vi "Dashboard Main.vi"() -> ()   [LabVIEW 2012]
uses:
  <vilib>/event_ctls.llb/eventvkey.ctl
  <vilib>/Utility/config.llb/Read Key (String).vi
  <vilib>/Utility/config.llb/Read Key (I32).vi
  <vilib>/Utility/config.llb/Write Key (String).vi
  <vilib>/Utility/config.llb/Write Key (I32).vi
  <vilib>/Utility/config.llb/NI_LVConfig.lvlib
panel:
  out "Decal 25":bool
  out "Decal 24":bool
  out "Decal 23":bool
  out "Decal 22":bool
  out "Decal 21":bool
  out "Decal 20":bool
  out "Decal 19":bool
  out "Decal 18":bool
  out "Decal 17":bool
  out "Decal 16":bool
  out "Decal 15":bool
  out "Decal 14":bool
  out "Decal 13":bool
  out "Decal 12":bool
  out "Decal 11":bool
  out "Decal 10":bool
  out "Decal 9":bool
  out "Decal 8":bool
  out "Decal 7":bool
  out "Decal 6":bool
  out "Decal 5":bool
  out "Decal 4":bool
  out "Decal 3":bool
  out "Decal 2":bool
  out "Decal 1":bool
  in  "Camera Settings":T1={"Frate Rate"=30, "Compression"=30, "Size"=1} {"Frate Rate" scale=1.0..30.0; "Size" items=["640x480", "320x240", "160x120"]}
  out "Mode":T2(ring)=enum."Auto Disabled"
  out "Camera IP":string
  in  "Dashboard Tab":enum32{"Operation", "Test", "Checklist"}(tab)
  out "Height":dbl format="%#_4g"
  out "Move Y":dbl format="%#_4g"
  out "Move X":dbl format="%#_4g"
  out "Rotation":dbl format="%#_4g"
  out "Min Height":bool
  out "Max Height":bool
  out "Feed Disc":bool
  in  "Set Launcher":dbl(slide) scale=0.0..100.0
  in  "Invert Motors":bool
  out "Rotation Output":dbl(knob) scale=0.0..100.0
  out "Linear Output":dbl(knob) scale=0.0..100.0
  out "Launcher Power":dbl(knob) scale=0.0..100.0
  out "Low Battery":bool
  out "FMS":bool
  out "Test":bool
  out "Teleop":bool
  out "Auto":bool
  out "Disabled":bool
  out "Program:":string caption="Program"
  out "Robot IP:":string caption="Robot IP"
  in  "Slider":dbl(slide) scale=0.0..100.0 scale format="%#_3g"
  in  "On/Off":bool caption="Solenoid"
  in  "Test Name":u16(ring) items=["Select the test to run...", "Example Test", "-------------------------------", "List of tests is built in robot code.", "Replace with your own automated tests."]
  in  "Test Tree":string(tree)
  in  "Motor":cluster{"Value":dbl, "Enable":bool} {"Value" scale=-1.0..1.0 scale format="%#_3g"}
  out "Progress":T3 {"Test Progress" scale=0.0..100.0}
  in  "Rev/Fwd":cluster{"Forward":bool, "Reverse":bool}
  in  "Ring":u16(ring) items=["Auto", "Fixed indoor", "Fixed outdoor 1", "Fixed outdoor 2", "Fixed fluorescent 1", "Fixed fluorescent 2", "Hold current"]
  in  "Listbox":i32(listbox)
  in  "Viewer":enum32{"Camera Image", "Variables"}(tab)
  in  "DB Camera Config":bool
  out "Mbps":dbl format="%#.1g"
  out "Mbps":bool
  in  "Enable":bool
  out "Image Error Message":string="Timeout in Camera Communications"
  out "Camera Image":T4(plugin-control)
  out "Tree":string(tree)
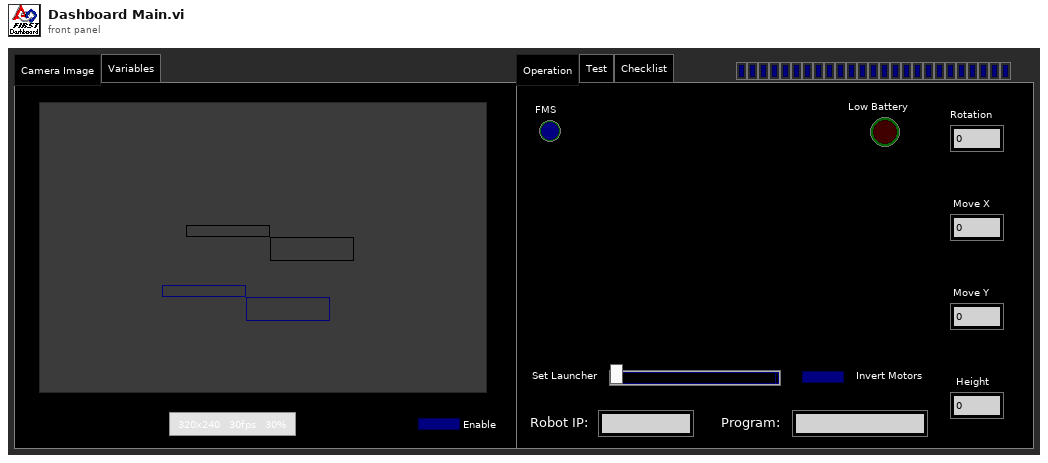
[diagram p1: front panel]
types:
  T1 = cluster{"Frate Rate":i32, "Compression":i32, "Size":u16}
  T2 = enum8{"Tele-Op Disabled", "Tele-Op Enabled", "Auto Disabled", "Auto Enabled", "Test Disabled", "Test Enabled", ""}
  T3 = cluster{"Test Progress":u8, "Test Progress Text":string}
  T4 = typedef "IMAQ Image.ctl" = refnum<image>
  T5 = typedef "Image Type" = u32
  T6 = typedef "SkeletonTrackState.ctl" = enum32{"NotTracked", "PositionOnly", "Tracked"}
  T7 = cluster{"TrackingState":u8[], "Position":cluster{"x":sgl, "y":sgl, "z":sgl}, cluster{"x":sgl, "y":sgl, "z":sgl, sgl}[], "TrackState":T6}
  T8 = cluster{cluster{"ScaledToPercentRange":dbl, "ScaledToPercentRange":dbl, "ScaledToPercentRange":dbl}, cluster{bool, bool, bool}}[]
  T9 = cluster{cluster{"ScaledToPercentRange":dbl, "ScaledToPercentRange":dbl, "ScaledToPercentRange":dbl}, cluster{bool, bool, bool}}
  T10 = typedef "LVRectTypeDef.ctl" = cluster{"Left":i16, "Top":i16, "Right":i16, "Bottom":i16}
  T11 = cluster{"Competition mode":bool, "Robot Link":bool, "Autonomous":bool, "Enabled":bool, "E-Stop":bool, "Simulated":bool, "TestMode":bool, "Docked Window":bool}
  T12 = typedef "NI_LVConfig.lvlib/Config Data RefNum.ctl" = refnum<k1>
  T13 = typedef "eventvkey.ctl" = enum16{"ASCII", "Enter", "Return", "Shift", "Ctrl", "Alt", "Cmd", "Opt", "Caps", "NumLock", "Clear", "Break", "Up", "Down", "Left", "Right", "Insert", "Delete", "Home", "End", "PageUp", "PageDown", "Escape", "Help", "Pause", "ScrollLock", "F1", "F2", "F3", "F4", "F5", "F6", "F7", "F8", "F9", "F10", "F11", "F12", "F13", "F14", "F15", "F16", "F17", "F18", "F19", "F20", "F21", "F22", "F23", "F24", "Play", "VolumeUp", "VolumeDown", "Mute", "Two Byte Char"}
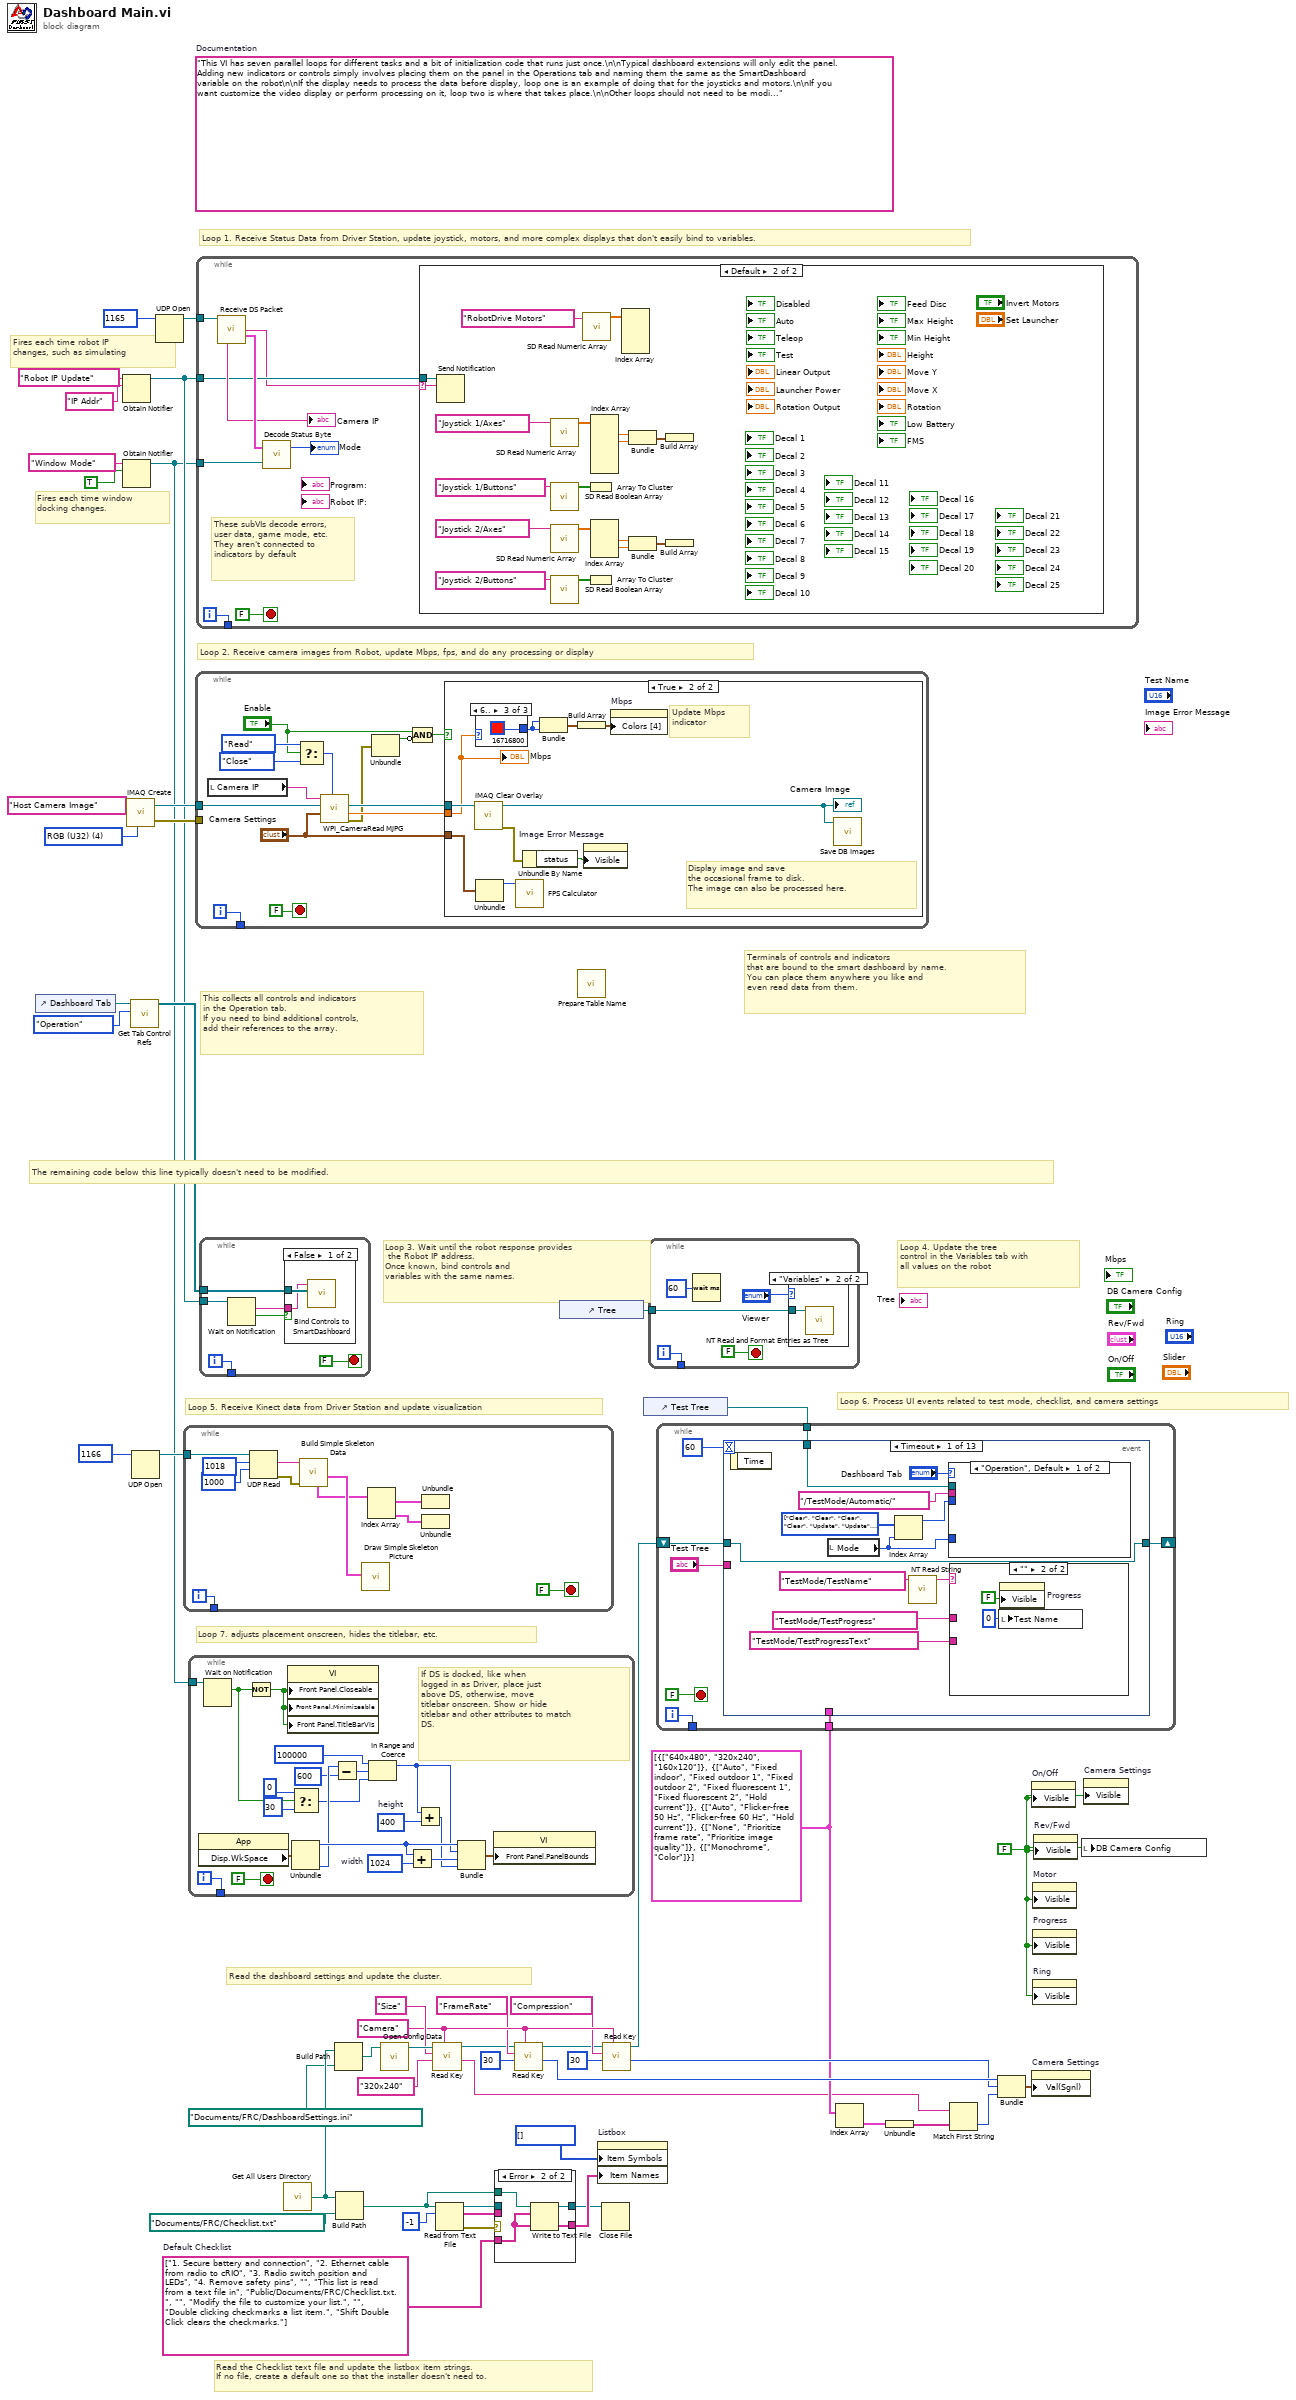
[diagram p0: block diagram]
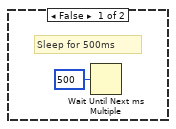
[diagram p3: hidden frame]
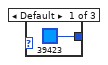
[diagram p4: hidden frame]
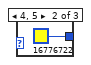
[diagram p5: hidden frame]
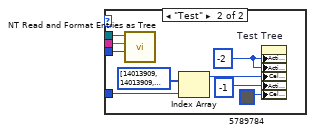
[diagram p7: hidden frame]
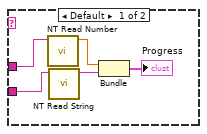
[diagram p8: hidden frame]
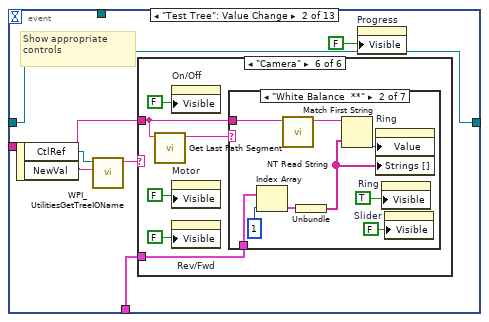
[diagram p9: hidden frame]
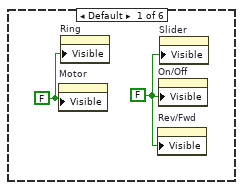
[diagram p10: hidden frame]
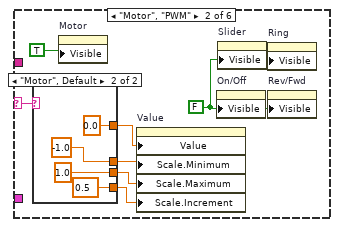
[diagram p11: hidden frame]
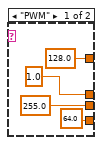
[diagram p12: hidden frame]
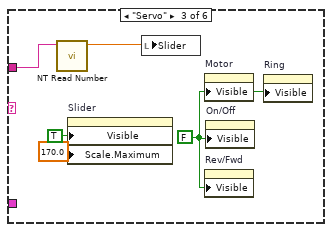
[diagram p13: hidden frame]
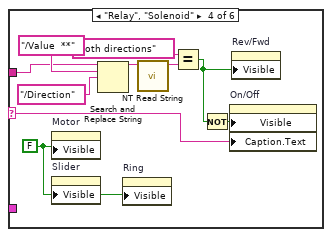
[diagram p14: hidden frame]
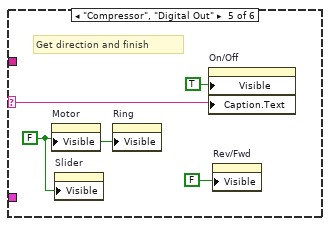
[diagram p15: hidden frame]
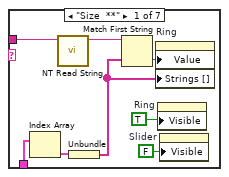
[diagram p16: hidden frame]
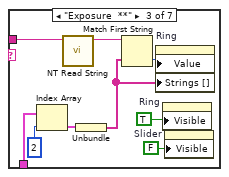
[diagram p17: hidden frame]
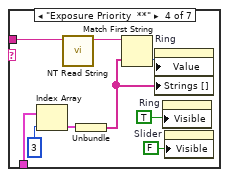
[diagram p18: hidden frame]
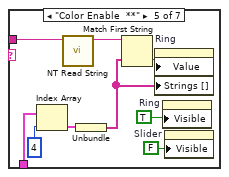
[diagram p19: hidden frame]
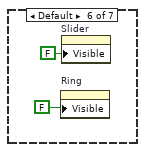
[diagram p20: hidden frame]
diagram:
  w21 = "Camera"
  w13 = cluster{string[]}[] [{["640x480", "320x240", "160x120"]}, {["Auto", "Fixed indoor", "Fixed outdoor 1", "Fixed outdoor 2", "Fixed fluorescent 1", "Fixed fluorescent 2", "Hold current"]}, {["Auto", "Flicker-free 50 Hz", "Flicker-free 60 Hz", "Hold current"]}, {["None", "Prioritize frame rate", "Prioritize image quality"]}, {["Monochrome", "Color"]}]
  w29 = string[] ["1. Secure battery and connection", "2. Ethernet cable from radio to cRIO", "3. Radio switch position and LEDs", "4. Remove safety pins", "", "This list is read from a text file in", "Public/Documents/FRC/Checklist.txt.", "", "Modify the file to customize your list.", "", "Double clicking checkmarks a list item.", "Shift Double Click clears the checkmarks."]  # Default Checklist
  w27 = FALSE ("Visible")
  (unwired) "This VI has seven parallel loops for different tasks and a bit of initialization code that runs just once.\n\nTypical dashboard extensions will only edit the panel. Adding new indicators or controls simply involves placing them on the panel in the Operations tab and naming them the same as the SmartDashboard variable on the robot\n\nIf the display needs to process the data before display, loop one is an example of doing that for the joysticks and motors.\n\nIf you want customize the video display or perform processing on it, loop two is where that takes place.\n\nOther loops should not need to be modified. They are pretty standard, and document the task they perform."  # Documentation
  w50 = T5 4 items=["Grayscale (U8)", "Grayscale (I16)", "Grayscale (SGL)", "Complex (CSG)", "RGB (U32)", "HSL (U32)", "RGB (U64)"] ("Image Type")
  # "Fires each time robot IP\nchanges, such as simulating"
  # "Fires each time window\ndocking changes."
  # "Read the Checklist text file and update the listbox item strings.\nIf no file, create a default one so that the installer doesn't need to."
  # "This collects all controls and indicators\nin the Operation tab.\nIf you need to bind additional controls,\nadd their references to the array."
  # "The remaining code below this line typically doesn't need to be modified."
  # "Loop 6. Process UI events related to test mode, checklist, and camera settings"
  # "Read the dashboard settings and update the cluster."
  # "Terminals of controls and indicators\nthat are bound to the smart dashboard by name.\nYou can place them anywhere you like and\neven read data from them."
  # "Loop 4. Update the tree\ncontrol in the Variables tab with\nall values on the robot"
  # "Loop 3. Wait until the robot response provides\n the Robot IP address.\nOnce known, bind controls and\nvariables with the same names."
  # "Loop 5. Receive Kinect data from Driver Station and update visualization"
  # "Loop 7. adjusts placement onscreen, hides the titlebar, etc."
  # "Loop 1. Receive Status Data from Driver Station, update joystick, motors, and more complex displays that don't easily bind to variables."
  # "Loop 2. Receive camera images from Robot, update Mbps, fps, and do any processing or display"
  n1 = control-ref of="Dashboard Tab"() -> (w43:refnum<vi>)
  n2 = Obtain Notifier(name (unnamed)="Robot IP Update", notification data type="IP Addr" ("name (unnamed)")) -> (notifier out=w40:refnum<notifier>)  [unwired: 2 in, 2 out]
  n3 = Obtain Notifier(name (unnamed)="Window Mode", notification data type=TRUE) -> (notifier out=w33:refnum<notifier>)  [unwired: 2 in, 2 out]
  n4 = call "IMAQ Create"("Image Name"="Host Camera Image", "Image Type"=w50) -> ("New Image"=w48:T4, "error out"=w47:errorcluster)  [unwired: 2 in, 1 out]
  n5 = call <vilib>:"Get Tab Control Refs.vi"("Page Index"=enum32{"Operation", "Test"}."Operation" ("Dashboard Tab"), "TabControl in"=w43) -> ("ControlsOnPage"=w44:refnum<vi>[])  [unwired: 9 in]
  n6 = UDP Open(11:u16 1166 ("port")) -> (port=w45:refnum<k16>)  [unwired: 2 in, 4 out]
  n7 = UDP Open(11:u16 1165 ("port")) -> (port=w51:refnum<k16>)  [unwired: 2 in, 4 out]
  n8 = while {
    tunnel: w45 -> [w61]
    tunnel: [w54] -> _
    i -> [w54]
    stop <- FALSE stop-if-true
    n9 = UDP Read(connection ID=w61, max size (548)=1018 ("bytes to read"), timeout ms (25000)=1000) -> (data out=w59:string, error out=w53:errorcluster)  [unwired: 1 in, 3 out]
    n10 = call "Build Simple Skeleton Data.vi"("error in (no error)"=w53, "data in"=w59) -> ("Skeleton Data"=w60:T7, "Simple Joystick Info"=w57:T8)  [unwired: 5 in, 3 out]
    n11 = call "Draw Simple Skeleton Picture.vi"("Simple Skeleton"=w60) -> ()  [unwired: 10 in, 1 out]
    n12 = Index Array(array=w57) -> (element #1=w56:T9, element #2=w55:T9)  [unwired: 2 in]
    n13 = Unbundle(w56) -> ()  [unwired: 2 out]
    n14 = Unbundle(w55) -> ()  [unwired: 2 out]
  }
  n15 = while {
    tunnel: w33 -> [w82]
    tunnel: [w80] -> _
    i -> [w80]
    stop <- FALSE stop-if-true
    w72 = 1024  # width
    w75 = 400  # height
    # "If DS is docked, like when\nlogged in as Driver, place just\nabove DS, otherwise, move\ntitlebar onscreen. Show or hide\ntitlebar and other attributes to match\nDS."
    n16 = property class="App"() -> ("Disp.WkSpace"=w78:T10)  [unwired: 2 in, 2 out]
    n17 = Wait on Notification(notifier=w82) -> (notification=w67:bool)  [unwired: 3 in, 3 out]
    n18 = Not(x=w67) -> (.not. x?=w81:bool)
    n19 = property class="VI"("Front Panel.Closeable"=w81, "Front Panel.Minimizeable"=w81, "Front Panel.TitleBarVis"=w81) -> ()  [unwired: 2 in, 2 out]
    n20 = Unbundle(w78) -> ("Left"=w76:i16, "Bottom"=w73:i16)  [unwired: 2 out]
    n21 = Select(t=0, s=w67, f=30) -> (s? t:f=w66:i32)
    n22 = Subtract(x=w73, y=600) -> (x-y=w70:i32)
    n23 = In Range and Coerce(upper limit=100000, x=w70, lower limit=w66) -> (coerced(x)=w64:i32)  [unwired: 1 out]
    n24 = Add(x=w76, y=w72) -> (x+y=w77:i32)
    n25 = Add(x=w64, y=w75) -> (x+y=w74:i32)
    n26 = Bundle("Left"=w76, w64, w77, w74) -> (w79:cluster{"Left":i16, i32, i32, i32})  [unwired: 1 out]
    n27 = property class="VI"("Front Panel.PanelBounds"=w79) -> ()  [unwired: 2 in, 2 out]
  }
  n28 = while {
    tunnel: w48 -> [w93]
    tunnel: w47 -> [_]
    tunnel: [w96] -> _
    i -> [w96]
    stop <- FALSE stop-if-true
    n29 = local read "Camera IP"() -> (w95:string)
    n30 = Select(t=enum16{"Read", "Reopen", "Close"}."Read" ("Operation"), s="Enable", f=enum16{"Read", "Reopen", "Close"}."Close" ("Operation")) -> (s? t:f=w88:enum16{"Read", "Reopen", "Close"})
    n31 = call <vilib>:"WPI_CameraRead MJPG.vi"("Operation"=w88, "Camera Settings"="Camera Settings", "Image"=w93, "address"=w95) -> ("error out"=w87:errorcluster, "Bandwidth (kbps)"=w91:dbl, "Image Out"=w92:T4)  [unwired: 5 in]
    n32 = Unbundle(w87) -> ("status"=w85:bool)  [unwired: 2 out]
    n33 = Compound Arithmetic op=AND("Enable", invert w85) -> (w84:bool)
    n34 = case shown="True" w84 {
      tunnel: "Camera Settings" -> [_ w100]
      tunnel: w92 -> [_ w102]
      tunnel: w91 -> [_ w101]
      frame False {
        # "Sleep for 500ms"
        n35 = Wait Until Next ms Multiple(millisecond multiple=u32 500) -> ()  [unwired: 1 out]
      }
      frame True {
        # "Display image and save\nthe occasional frame to disk.\nThe image can also be processed here."
        # "Update Mbps\nindicator"
        n36 = call "IMAQ Clear Overlay"("Image"=w102) -> ("error out"=w107:errorcluster, "Image Out"=w106:T4)  [unwired: 2 in, 7 out]
        "Camera Image" <- w106
        n37 = case shown="6.." w101 {
          tunnel: [u32 39423 ("Color Box") u32 16776722 ("Color Box") u32 16716800 ("Color Box")] -> w103
          frame Default {
          }
          frame 4, 5 {
          }
          frame 6.. {
          }
        }
        n38 = Unbundle(w100) -> ("Frate Rate"=w99:i32)  [unwired: 2 out]
        n39 = call "FPS Calculator.vi"("Average Count"=w99) -> ()  [unwired: 10 in, 1 out]
        n40 = Unbundle By Name(w107) -> ("status"=w108:bool)
        n41 = Bundle("Color Box"=w103, "Color Box"=w103) -> (w105:cluster{"Color Box":u32, "Color Box":u32})  [unwired: 1 out]
        n42 = Build Array(w105) -> (w104:cluster{"Color Box":u32, "Color Box":u32}[])
        n43 = property on="Image Error Message" class="Str"("Visible"=w108) -> ()  [unwired: 2 in, 2 out]
        n44 = property on="Mbps" class="Bool (strict)"("Colors [4]"=w104) -> ()  [unwired: 2 in, 2 out]
        n45 = call "Save DB Images.vi"("Image"=w106) -> ()  [unwired: 2 in, 1 out]
        "Mbps" <- w101
      }
    }
  }
  n46 = while {
    tunnel: w51 -> [w118]
    tunnel: w40 -> [w113]
    tunnel: w33 -> [w117]
    tunnel: [w114] -> _
    i -> [w114]
    stop <- FALSE stop-if-true
    # "These subVIs decode errors, user data, game mode, etc.\nThey aren't connected to indicators by default"
    n47 = call "Receive DS Packet.vi"("Recv Socket"=w118) -> ("Robot IP Address"=w112:string, "Status"=w119:T11, "Camera IP Address"=→"Camera IP":string)  [unwired: 1 in, 11 out]
    n48 = call "Decode Status Byte.vi"("Window Mode Notifier"=w117, "Status"=w119) -> ("Mode"=→"Mode":T2)  [unwired: 1 out]
    n49 = case shown="Default" w112 {
      selector: w112 -> [_ w121]
      tunnel: w113 -> [_ w122]
      frame "0.0.0.0" {
        # "Robot not responding, don't poll the variables"
      }
      frame Default {
        n50 = Send Notification(notification=w121, notifier=w122) -> ()  [unwired: 1 in, 2 out]
        n51 = call <vilib>:"SD Read Numeric Array.vi"("Name"="Joystick 1/Axes") -> ("Numeric Array"=w133:dbl[])  [unwired: 8 in, 2 out]
        n52 = call <vilib>:"SD Read Boolean Array.vi"("Name"="Joystick 1/Buttons") -> ("Boolean Array"=w134:bool[])  [unwired: 8 in, 2 out]
        n53 = call <vilib>:"SD Read Numeric Array.vi"("Name"="Joystick 2/Axes") -> ("Numeric Array"=w129:dbl[])  [unwired: 8 in, 2 out]
        n54 = call <vilib>:"SD Read Boolean Array.vi"("Name"="Joystick 2/Buttons") -> ("Boolean Array"=w128:bool[])  [unwired: 8 in, 2 out]
        n55 = call <vilib>:"SD Read Numeric Array.vi"("Name"="RobotDrive Motors") -> ("Numeric Array"=w135:dbl[])  [unwired: 8 in, 2 out]
        n56 = Array To Cluster(array=w134) -> ()  [unwired: 1 out]
        n57 = Array To Cluster(array=w128) -> ()  [unwired: 1 out]
        n58 = Index Array(array=w133) -> (element #1=w131:dbl, element #2=w132:dbl)  [unwired: 6 in, 4 out]
        n59 = Index Array(array=w129) -> (element #1=w124:dbl, element #2=w123:dbl)  [unwired: 3 in, 1 out]
        n60 = Index Array(array=w135) -> ()  [unwired: 4 in, 4 out]
        n61 = Bundle("Numeric"=w131, "Numeric"=w132) -> (w130:cluster{"Numeric":dbl, "Numeric":dbl})  [unwired: 1 in]
        n62 = Bundle("Numeric"=w124, "Numeric"=w123) -> (w125:cluster{"Numeric":dbl, "Numeric":dbl})  [unwired: 1 in]
        n63 = Build Array(w130) -> ()  [unwired: 1 out]
        n64 = Build Array(w125) -> ()  [unwired: 1 out]
      }
    }
  }
  n65 = while {
    tunnel: w44 -> [w144]
    tunnel: w40 -> [w141]
    tunnel: [w139] -> _
    i -> [w139]
    stop <- FALSE stop-if-true
    n66 = Wait on Notification(notifier=w141) -> (notification=w140:string, timed out?=w142:bool)  [unwired: 3 in, 2 out]
    n67 = case shown="False" w142 {
      tunnel: w144 -> [w146 _]
      tunnel: w140 -> [w145 _]
      frame False {
        n68 = call <vilib>:"Bind Controls to SmartDashboard.vi"("Bound Control Refs"=w146, "Server IP Address"=w145) -> ()  [unwired: 10 in]
      }
      frame True {
      }
    }
  }
  n69 = call "Get All Users Directory.vi"() -> ("All User Path"=w26:path)
  n70 = Build Path(base path=w26, name or relative path=path "Documents/FRC/DashboardSettings.ini") -> (appended path=w25:path)
  n71 = Build Path(base path=w26, name or relative path=path "Documents/FRC/Checklist.txt") -> (appended path=w30:path)
  n72 = call <vilib>:"Open Config Data.vi"("configuration file path"=w25) -> ("refnum"=w24:T12)  [unwired: 8 in, 2 out]
  n73 = call-poly <vilib>:"Read Key.vi"("section"=w21, "default value"="320x240", "key"="Size", "refnum"=w24) -> ("value"=w11:string, "refnum out"=w6:T12)  [unwired: 2 in, 4 out]
  n74 = Read from Text File(file (use dialog)=w30, count=-1 ("timeout ms (25000)")) -> (refnum out=w8:refnum<file>, text=w31:string[], error out=w32:errorcluster)  [unwired: 2 in, 1 out]
  n75 = case shown="Error" w32 {
    tunnel: w31 -> [w148 _]
    tunnel: [w148 w150] -> w28
    tunnel: w29 -> [_ w150]
    tunnel: w30 -> [_ w151]
    tunnel: [w147 w149] -> w7
    tunnel: w8 -> [w147 _]
    frame No Error {
    }
    frame Error {
      n76 = Write to Text File(file (use dialog)=w151, text=w150) -> (refnum out=w149:refnum<file>)  [unwired: 2 in, 2 out]
    }
  }
  n77 = call-poly <vilib>:"Read Key.vi"("section"=w21, "default value"=30, "key"="FrameRate", "refnum"=w6) -> ("value"=w16:i32, "refnum out"=w5:T12)  [unwired: 1 in, 5 out]
  n78 = control-ref of="Tree"() -> (w2:refnum<vi>)
  n79 = call <vilib>:"Prepare Table Name.vi"() -> ()  [unwired: 11 in, 1 out]
  n80 = property on="Listbox" class="LstBox (strict)"("Item Symbols"=i32[] [], "Item Names"=w28) -> ()  [unwired: 2 in, 2 out]
  n81 = Close File(refnum=w7) -> ()  [unwired: 1 in, 2 out]
  n82 = call-poly <vilib>:"Read Key.vi"("section"=w21, "default value"=30, "key"="Compression", "refnum"=w5) -> ("value"=w15:i32, "refnum out"=w3:T12)  [unwired: 1 in, 5 out]
  n83 = control-ref of="Test Tree"() -> (w1:refnum<vi>)
  n84 = while {
    tunnel: [w153] -> _
    tunnel: w2 -> [w152]
    i -> [w153]
    stop <- FALSE stop-if-true
    n85 = Wait (ms)(milliseconds to wait=u32 60) -> ()  [unwired: 1 out]
    n86 = case shown="\"Variables\"" "Viewer" {
      tunnel: w152 -> [_ w157]
      frame Default {
      }
      frame "Variables" {
        n87 = call <vilib>:"NT Read and Format Entries as Tree.vi"("Tree Refnum"=w157) -> ()  [unwired: 9 in, 2 out]
      }
    }
  }
  n88 = while {
    tunnel: w13 -> [w162]
    shift-right: [w161] -> _
    shift-left: w3 -> [w160]
    tunnel: [w159] -> _
    tunnel: w1 -> [w158]
    i -> [w159]
    stop <- FALSE stop-if-true
    n89 = event shown="[0] Timeout" {
      selector: _ -> [_ _ _ _ _ _ _ _ _ _ _ _ _]
      dyn-events: _ -> [_ _ _ _ _ _ _ _ _ _ _ _ _]
      timeout: u32 60 ("milliseconds to wait") -> [_ _ _ _ _ _ _ _ _ _ _ _ _]
      tunnel: w158 -> [w172 _ _ _ _ _ _ _ _ _ _ _ _]
      tunnel: "Test Tree" -> [_ _ _ _ _ _ _ _ w366 w374 w376 w380 w388]
      tunnel: w162 -> [_ w194 _ _ _ _ w330 w360 _ _ _ _ _]
      tunnel: [w166 w193 _ w296 w304 w316 w329 w353 w365 w372 w375 w379 w387] -> w161
      tunnel: w160 -> [w166 w193 _ w296 w304 w316 w328 w353 w365 w372 w375 w379 w387]
      event Timeout {
        w171 = enum16{"Update", "Clear"}[] [enum."Clear", enum."Clear", enum."Clear", enum."Clear", enum."Update", enum."Update", enum."Clear"] items=["Update", "Clear"]
        n90 = event-data() -> ()  [unwired: 1 in, 1 out]
        n91 = local read "Mode"() -> (w169:T2)
        n92 = Index Array(array=w171, index=w169) -> (element=w170:enum16{"Update", "Clear"})
        n93 = call <vilib>:"NT Read String.vi"("Name"="TestMode/TestName") -> ("String"=w175:string)  [unwired: 9 in, 1 out]
        n94 = case shown="\"Operation\", Default" "Dashboard Tab" {
          tunnel: w172 -> [_ w185]
          tunnel: "/TestMode/Automatic/" ("Name Pattern") -> [_ w184]
          tunnel: w170 -> [_ w183]
          tunnel: w169 -> [_ w181]
          frame "Operation", Default {
          }
          frame "Test" {
            w180 = -2 ("Active Item:Row Number")
            n95 = call <vilib>:"NT Read and Format Entries as Tree.vi"("Operation"=w183, "Name Pattern"=w184, "Tree Refnum"=w185) -> ()  [unwired: 7 in, 2 out]
            n96 = Index Array(array=u32[] [14013909, 14013909, 14013909, 14013909, 14013909, 16777215, 14013909], index=w181) -> (element=w179:u32)
            n97 = property on="Test Tree" class="Tree (strict)"("Active Item Row Number"=w180, "ActiveColNum"=w180, "CellBG"=w179, "Active Item Row Number"=-1 ("Active Item:Row Number"), "CellBG"=u32 5789784 ("Color Box")) -> ()  [unwired: 2 in, 2 out]
          }
        }
        n98 = case shown="\"\"" w175 {
          tunnel: "TestMode/TestProgress" ("Name") -> [w187 _]
          tunnel: "TestMode/TestProgressText" ("Name") -> [w186 _]
          frame Default {
            n99 = call <vilib>:"NT Read Number.vi"("Name"=w187) -> ("Numeric"=w188:dbl)  [unwired: 9 in, 1 out]
            n100 = call <vilib>:"NT Read String.vi"("Name"=w186) -> ("String"=w189:string)  [unwired: 9 in, 1 out]
            n101 = Bundle("Numeric"=w188, "String"=w189) -> (→"Progress":cluster{"Numeric":dbl, "String":string})  [unwired: 1 in]
          }
          frame "" {
            n102 = local write "Test Name"(u16 0) -> ()
            n103 = property on="Progress" class="Clust (strict)"("Visible"=FALSE) -> ()  [unwired: 2 in, 2 out]
          }
        }
      }
      event "Test Tree": Value Change {
        # "Show appropriate\ncontrols"
        n104 = event-data() -> ("CtlRef"=w197:refnum<vi>, "NewVal"=w195:string)  [unwired: 1 in]
        n105 = call <vilib>:"WPI_UtilitiesGetTreeIOName.vi"("NewVal"=w195, "TreeControl in"=w197) -> ("I/O Name"=w198:string)  [unwired: 9 in]
        n106 = case shown="\"Camera\"" w198 {
          selector: w198 -> [_ w205 _ w223 w232 _]
          tunnel: w195 -> [_ _ w220 w222 _ w239]
          tunnel: w194 -> [_ _ _ _ _ w238]
          frame Default {
            w200 = FALSE ("Visible")
            w199 = FALSE ("Visible")
            n107 = property on="Motor" class="Clust (strict)"("Visible"=w199) -> ()  [unwired: 2 in, 2 out]
            n108 = property on="Ring" class="Ring (strict)"("Visible"=w199) -> ()  [unwired: 2 in, 2 out]
            n109 = property on="Rev/Fwd" class="Clust (strict)"("Visible"=w200) -> ()  [unwired: 2 in, 2 out]
            n110 = property on="On/Off" class="Bool (strict)"("Visible"=w200) -> ()  [unwired: 2 in, 2 out]
            n111 = property on="Slider" class="Slide (strict)"("Visible"=w200) -> ()  [unwired: 2 in, 2 out]
          }
          frame "Motor", "PWM" {
            w206 = FALSE ("Visible")
            n112 = case shown="\"Motor\", Default" w205 {
              tunnel: [1.0 ("Value") -1.0 ("Value")] -> w204
              tunnel: [255.0 ("Value") 1.0 ("Value")] -> w203
              tunnel: [128.0 ("Value") 0.0 ("Value")] -> w202
              tunnel: [64.0 ("Value") 0.5 ("Value")] -> w201
              frame "PWM" {
              }
              frame "Motor", Default {
              }
            }
            n113 = property on="Motor" class="Clust (strict)"("Visible"=TRUE) -> ()  [unwired: 2 in, 2 out]
            n114 = property on="Value" class="Slide (strict)"("Value"=w202, "Scale.Minimum"=w204, "Scale.Maximum"=w203, "Scale.Increment"=w201) -> ()  [unwired: 2 in, 2 out]
            n115 = property on="On/Off" class="Bool (strict)"("Visible"=w206) -> ()  [unwired: 2 in, 2 out]
            n116 = property on="Slider" class="Slide (strict)"("Visible"=w206) -> ()  [unwired: 2 in, 2 out]
            n117 = property on="Ring" class="Ring (strict)"("Visible"=w206) -> ()  [unwired: 2 in, 2 out]
            n118 = property on="Rev/Fwd" class="Clust (strict)"("Visible"=w206) -> ()  [unwired: 2 in, 2 out]
          }
          frame "Servo" {
            w218 = FALSE ("Visible")
            n119 = call <vilib>:"NT Read Number.vi"("Name"=w220) -> ("Numeric"=w219:dbl)  [unwired: 9 in, 1 out]
            n120 = property on="Slider" class="Slide (strict)"("Visible"=TRUE, "Scale.Maximum"=170.0 ("Scale.Range:Maximum")) -> ()  [unwired: 2 in, 2 out]
            n121 = local write "Slider"(w219) -> ()
            n122 = property on="Motor" class="Clust (strict)"("Visible"=w218) -> ()  [unwired: 2 in, 2 out]
            n123 = property on="Rev/Fwd" class="Clust (strict)"("Visible"=w218) -> ()  [unwired: 2 in, 2 out]
            n124 = property on="On/Off" class="Bool (strict)"("Visible"=w218) -> ()  [unwired: 2 in, 2 out]
            n125 = property on="Ring" class="Ring (strict)"("Visible"=w218) -> ()  [unwired: 2 in, 2 out]
          }
          frame "Relay", "Solenoid" {
            w221 = FALSE ("Visible")
            n126 = property on="Motor" class="Clust (strict)"("Visible"=w221) -> ()  [unwired: 2 in, 2 out]
            n127 = property on="Slider" class="Slide (strict)"("Visible"=w221) -> ()  [unwired: 2 in, 2 out]
            n128 = Search and Replace String(input string=w222, search string="/Value  **", replace string="/Direction") -> (result string=w228:string)  [unwired: 5 in, 3 out]
            n129 = property on="Ring" class="Ring (strict)"("Visible"=w221) -> ()  [unwired: 2 in, 2 out]
            n130 = call <vilib>:"NT Read String.vi"("Name"=w228) -> ("String"=w226:string)  [unwired: 9 in, 1 out]
            n131 = Equal?(x="Both directions", y=w226) -> (x = y?=w224:bool)
            n132 = Not(x=w224) -> (.not. x?=w225:bool)
            n133 = property on="On/Off" class="Bool (strict)"("Visible"=w225, "Caption.Text"=w223) -> ()  [unwired: 2 in, 2 out]
            n134 = property on="Rev/Fwd" class="Clust (strict)"("Visible"=w224) -> ()  [unwired: 2 in, 2 out]
          }
          frame "Compressor", "Digital Out" {
            w231 = FALSE ("Visible")
            # "Get direction and finish"
            n135 = property on="Motor" class="Clust (strict)"("Visible"=w231) -> ()  [unwired: 2 in, 2 out]
            n136 = property on="Slider" class="Slide (strict)"("Visible"=w231) -> ()  [unwired: 2 in, 2 out]
            n137 = property on="Ring" class="Ring (strict)"("Visible"=w231) -> ()  [unwired: 2 in, 2 out]
            n138 = property on="On/Off" class="Bool (strict)"("Visible"=TRUE, "Caption.Text"=w232) -> ()  [unwired: 2 in, 2 out]
            n139 = property on="Rev/Fwd" class="Clust (strict)"("Visible"=FALSE) -> ()  [unwired: 2 in, 2 out]
          }
          frame "Camera" {
            n140 = call <vilib>:"Get Last Path Segment.vi"("String in"=w239) -> ("String out"=w240:string)  [unwired: 10 in]
            n141 = property on="On/Off" class="Bool (strict)"("Visible"=FALSE) -> ()  [unwired: 2 in, 2 out]
            n142 = property on="Motor" class="Clust (strict)"("Visible"=FALSE) -> ()  [unwired: 2 in, 2 out]
            n143 = property on="Rev/Fwd" class="Clust (strict)"("Visible"=FALSE) -> ()  [unwired: 2 in, 2 out]
            n144 = case shown="\"White Balance  **\"" w240 {
              tunnel: w239 -> [w246 w255 w264 w273 w282 _ w288]
              tunnel: w238 -> [w244 w252 w261 w270 w279 _ _]
              frame "Size  **" {
                n145 = Index Array(array=w244) -> (element=w243:cluster{string[]})  [unwired: 1 in]
                n146 = call <vilib>:"NT Read String.vi"("Name"=w246) -> ("String"=w245:string)  [unwired: 9 in, 1 out]
                n147 = Unbundle(w243) -> (w241:string[])
                n148 = Match First String(2:w241, 3:w245) -> (0:w242:i32)  [unwired: 1 out]
                n149 = property on="Ring" class="Ring (strict)"("Value"=w242, "Strings []"=w241) -> ()  [unwired: 2 in, 2 out]
                n150 = property on="Ring" class="Ring (strict)"("Visible"=TRUE) -> ()  [unwired: 2 in, 2 out]
                n151 = property on="Slider" class="Slide (strict)"("Visible"=FALSE) -> ()  [unwired: 2 in, 2 out]
              }
              frame "White Balance  **" {
                n152 = Index Array(array=w252, index=1) -> (element=w253:cluster{string[]})
                n153 = call <vilib>:"NT Read String.vi"("Name"=w255) -> ("String"=w254:string)  [unwired: 9 in, 1 out]
                n154 = Unbundle(w253) -> (w250:string[])
                n155 = Match First String(2:w250, 3:w254) -> (0:w249:i32)  [unwired: 1 out]
                n156 = property on="Ring" class="Ring (strict)"("Value"=w249, "Strings []"=w250) -> ()  [unwired: 2 in, 2 out]
                n157 = property on="Ring" class="Ring (strict)"("Visible"=TRUE) -> ()  [unwired: 2 in, 2 out]
                n158 = property on="Slider" class="Slide (strict)"("Visible"=FALSE) -> ()  [unwired: 2 in, 2 out]
              }
              frame "Exposure  **" {
                n159 = Index Array(array=w261, index=2) -> (element=w262:cluster{string[]})
                n160 = call <vilib>:"NT Read String.vi"("Name"=w264) -> ("String"=w263:string)  [unwired: 9 in, 1 out]
                n161 = Unbundle(w262) -> (w258:string[])
                n162 = Match First String(2:w258, 3:w263) -> (0:w259:i32)  [unwired: 1 out]
                n163 = property on="Ring" class="Ring (strict)"("Value"=w259, "Strings []"=w258) -> ()  [unwired: 2 in, 2 out]
                n164 = property on="Ring" class="Ring (strict)"("Visible"=TRUE) -> ()  [unwired: 2 in, 2 out]
                n165 = property on="Slider" class="Slide (strict)"("Visible"=FALSE) -> ()  [unwired: 2 in, 2 out]
              }
              frame "Exposure Priority  **" {
                n166 = Index Array(array=w270, index=3) -> (element=w271:cluster{string[]})
                n167 = call <vilib>:"NT Read String.vi"("Name"=w273) -> ("String"=w272:string)  [unwired: 9 in, 1 out]
                n168 = Unbundle(w271) -> (w267:string[])
                n169 = Match First String(2:w267, 3:w272) -> (0:w268:i32)  [unwired: 1 out]
                n170 = property on="Ring" class="Ring (strict)"("Value"=w268, "Strings []"=w267) -> ()  [unwired: 2 in, 2 out]
                n171 = property on="Ring" class="Ring (strict)"("Visible"=TRUE) -> ()  [unwired: 2 in, 2 out]
                n172 = property on="Slider" class="Slide (strict)"("Visible"=FALSE) -> ()  [unwired: 2 in, 2 out]
              }
              frame "Color Enable  **" {
                n173 = Index Array(array=w279, index=4) -> (element=w280:cluster{string[]})
                n174 = call <vilib>:"NT Read String.vi"("Name"=w282) -> ("String"=w281:string)  [unwired: 9 in, 1 out]
                n175 = Unbundle(w280) -> (w276:string[])
                n176 = Match First String(2:w276, 3:w281) -> (0:w277:i32)  [unwired: 1 out]
                n177 = property on="Ring" class="Ring (strict)"("Value"=w277, "Strings []"=w276) -> ()  [unwired: 2 in, 2 out]
                n178 = property on="Ring" class="Ring (strict)"("Visible"=TRUE) -> ()  [unwired: 2 in, 2 out]
                n179 = property on="Slider" class="Slide (strict)"("Visible"=FALSE) -> ()  [unwired: 2 in, 2 out]
              }
              frame Default {
                n180 = property on="Ring" class="Ring (strict)"("Visible"=FALSE) -> ()  [unwired: 2 in, 2 out]
                n181 = property on="Slider" class="Slide (strict)"("Visible"=FALSE) -> ()  [unwired: 2 in, 2 out]
              }
              frame "Brightness  **", "Color Level  **", "Compression  **", "FPS  **", "Sharpness  **" {
                n182 = call <vilib>:"NT Read Number.vi"("Name"=w288) -> ("Numeric"=w287:dbl)  [unwired: 9 in, 1 out]
                n183 = local write "Slider"(w287) -> ()
                n184 = property on="Slider" class="Slide (strict)"("Visible"=TRUE, "Scale.Maximum"=100.0 ("Scale.Range:Maximum")) -> ()  [unwired: 2 in, 2 out]
                n185 = property on="Ring" class="Ring (strict)"("Visible"=FALSE) -> ()  [unwired: 2 in, 2 out]
              }
            }
          }
        }
        n186 = property on="Progress" class="Clust (strict)"("Visible"=FALSE) -> ()  [unwired: 2 in, 2 out]
      }
      event "Test Name": Mouse Enter {
        # "Populate the ring with the list of tests"
        n187 = event-data() -> ()  [unwired: 1 in, 1 out]
        n188 = call <vilib>:"NT Read String Array.vi"("Name"="TestMode/TestList") -> ("String Array"=w295:string[])  [unwired: 9 in, 1 out]
        n189 = Build Array (concatenate)("Select the test to run...", w295) -> (w294:string[])
        n190 = property on="Test Name" class="Ring (strict)"("Strings []"=w294) -> ()  [unwired: 2 in, 2 out]
      }
      event "Test Name": Value Change {
        w297 = FALSE ("Visible")
        # "Tell the robot the test name to run"
        n191 = event-data() -> ("NewVal"=w301:u16)  [unwired: 1 in]
        n192 = property on="Test Name" class="Ring (strict)"() -> ("Strings []"=w302:string[])  [unwired: 2 in, 2 out]
        n193 = local write "Progress"(T3 {"Test Progress"=0, "Test Progress Text"=""} ("Progress")) -> ()
        n194 = Index Array(array=w302, index=w301) -> (element=w300:string)
        n195 = call <vilib>:"NT Write String.vi"("String"=w300, "Name"="TestMode/TestName") -> ()  [unwired: 9 in, 1 out]
        n196 = property on="Progress" class="Clust (strict)"("Visible"=TRUE) -> ()  [unwired: 2 in, 2 out]
        n197 = property on="Motor" class="Clust (strict)"("Visible"=w297) -> ()  [unwired: 2 in, 2 out]
        n198 = property on="Slider" class="Slide (strict)"("Visible"=w297) -> ()  [unwired: 2 in, 2 out]
        n199 = property on="On/Off" class="Bool (strict)"("Visible"=w297) -> ()  [unwired: 2 in, 2 out]
        n200 = property on="Rev/Fwd" class="Clust (strict)"("Visible"=w297) -> ()  [unwired: 2 in, 2 out]
        n201 = property on="Ring" class="Ring (strict)"("Visible"=w297) -> ()  [unwired: 2 in, 2 out]
      }
      event "Listbox": Double Click {
        n202 = event-data() -> ("PlatMods.Shift"=w305:bool, "Row"=w307:i32)  [unwired: 1 in]
        n203 = case shown="False" w305 {
          tunnel: w307 -> [w311 _]
          tunnel: 1 -> [w310 _]
          frame False {
            n204 = property on="Listbox" class="LstBox (strict)"() -> ("Item Symbols"=w309:i32[])  [unwired: 2 in, 2 out]
            n205 = Replace Array Subset(array=w309, new element=w310, index=w311) -> (w308:i32[])
            n206 = property on="Listbox" class="LstBox (strict)"("Item Symbols"=w308) -> ()  [unwired: 2 in, 2 out]
          }
          frame True {
            w312 = 0 ("Top Row")
            n207 = property on="Listbox" class="LstBox (strict)"() -> ("Number of Rows"=w314:u32)  [unwired: 2 in, 2 out]
            n208 = Initialize Array(0, w314) -> (w313:i32[])
            n209 = property on="Listbox" class="LstBox (strict)"("Top Row"=w312, "Value"=w312, "Item Symbols"=w313) -> ()  [unwired: 2 in, 2 out]
          }
        }
      }
      event "Listbox": Key Down {
        n210 = event-data() -> ("VKey"=w318:T13)  [unwired: 1 in]
        n211 = case shown="\"Left\", \"Right\"" w318 {
          selector: w318 -> [w323 _]
          tunnel: eventvkey."Left" ("VKey") -> [w321 _]
          frame "Left", "Right" {
            n212 = Equal?(x=w321, y=w323) -> (x = y?=w322:bool)
            n213 = Select(t=0, s=w322, f=1) -> (s? t:f=w324:i32)
            n214 = property on="Listbox" class="LstBox (strict)"() -> ("Item Symbols"=w327:i32[])  [unwired: 2 in, 2 out]
            n215 = Replace Array Subset(array=w327, new element=w324, index="Listbox") -> (w326:i32[])
            n216 = property on="Listbox" class="LstBox (strict)"("Item Symbols"=w326) -> ()  [unwired: 2 in, 2 out]
          }
          frame Default {
          }
        }
      }
      event "DB Camera Config": Value Change {
        n217 = event-data() -> ("NewVal"=w331:bool)  [unwired: 1 in]
        n218 = case shown="False" w331 {
          tunnel: w330 -> [w340 _]
          tunnel: [w333 w351] -> w329
          tunnel: w328 -> [w332 w351]
          frame False {
            w347 = "Camera"
            w350 = FALSE ("Visible")
            n219 = local read "Camera Settings"() -> (w339:T1)
            n220 = Index Array(array=w340) -> (element=w343:cluster{string[]})  [unwired: 1 in]
            n221 = Unbundle(w339) -> ("Frate Rate"=w338:i32, "Compression"=w337:i32, "Size"=w341:u16)
            n222 = Unbundle(w343) -> (w342:string[])
            n223 = Index Array(array=w342, index=w341) -> (element=w336:string)
            n224 = call-poly <vilib>:"Write Key.vi"("section"=w347, "value"=w336, "key"="Size", "refnum"=w332) -> ("refnum out"=w349:T12)  [unwired: 2 in, 5 out]
            n225 = call-poly <vilib>:"Write Key.vi"("section"=w347, "value"=w338, "key"="FrameRate", "refnum"=w349) -> ("refnum out"=w348:T12)  [unwired: 1 in, 6 out]
            n226 = local write "DB Camera Config"(w350) -> ()
            n227 = property on="Camera Settings" class="Clust (strict)"("Visible"=w350) -> ()  [unwired: 2 in, 2 out]
            n228 = call-poly <vilib>:"Write Key.vi"("section"=w347, "value"=w337, "key"="Compression", "refnum"=w348) -> ("refnum out"=w334:T12)  [unwired: 1 in, 6 out]
            n229 = call <vilib>:"Close Config Data.vi"("refnum"=w334) -> ("file path"=w335:path)  [unwired: 2 in, 8 out]
            n230 = call <vilib>:"Open Config Data.vi"("configuration file path"=w335) -> ("refnum"=w333:T12)  [unwired: 8 in, 2 out]
          }
          frame True {
            n231 = property on="Camera Settings" class="Clust (strict)"("Visible"=TRUE) -> ()  [unwired: 2 in, 2 out]
          }
        }
      }
      event "Camera Settings": Value Change {
        n232 = event-data() -> ("NewVal"=w364:T1)  [unwired: 1 in]
        n233 = Index Array(array=w360) -> (element=w359:cluster{string[]})  [unwired: 1 in]
        n234 = Unbundle(w364) -> ("Frate Rate"=w355:i32, "Compression"=w354:i32, "Size"=w357:u16)
        n235 = Unbundle(w359) -> (w358:string[])
        n236 = Index Array(array=w358, index=w357) -> (element=w356:string)
        n237 = Format Into String(format string="%s   %dfps   %d%%", w356, w355, w354) -> (resulting string=w361:string)  [unwired: 2 in, 1 out]
        n238 = Build Array(w361) -> (w362:string[])
        n239 = property on="DB Camera Config" class="Bool (strict)"("Strings [4]"=w362) -> ()  [unwired: 2 in, 2 out]
      }
      event "Motor.Enable": Value Change {
        n240 = event-data() -> ("NewVal"=w370:bool)  [unwired: 1 in]
        n241 = Unbundle("Motor") -> ("Value"=w369:dbl)  [unwired: 1 out]
        n242 = Select(t=w369, s=w370, f=0.0) -> (s? t:f=w367:dbl)
        n243 = call <vilib>:"NT Write Number.vi"("Numeric"=w367, "Name"=w366) -> ()  [unwired: 9 in, 1 out]
      }
      event "Slider": Value Change {
        n244 = event-data() -> ("NewVal"=w373:dbl)  [unwired: 1 in]
        n245 = call <vilib>:"NT Write Number.vi"("Numeric"=w373, "Name"=w374) -> ()  [unwired: 9 in, 1 out]
      }
      event "On/Off": Value Change {
        n246 = event-data() -> ("NewVal"=w378:bool)  [unwired: 1 in]
        n247 = Boolean To (0,1)(Boolean=w378) -> (0, 1=w377:i16)
        n248 = call <vilib>:"NT Write Number.vi"("Numeric"=w377, "Name"=w376) -> ()  [unwired: 9 in, 1 out]
      }
      event "Rev/Fwd": Value Change {
        n249 = event-data() -> ("NewVal.Forward"=w386:bool, "NewVal.Reverse"=w385:bool)  [unwired: 1 in]
        n250 = Boolean To (0,1)(Boolean=w386) -> (0, 1=w382:i16)
        n251 = Boolean To (0,1)(Boolean=w385) -> (0, 1=w384:i16)
        n252 = Negate(x=w384) -> (-x=w383:i16)
        n253 = Add(x=w382, y=w383) -> (x+y=w381:i16)
        n254 = call <vilib>:"NT Write Number.vi"("Numeric"=w381, "Name"=w380) -> ()  [unwired: 9 in, 1 out]
      }
      event "Ring": Value Change {
        n255 = event-data() -> ("NewVal"=w390:u16)  [unwired: 1 in]
        n256 = property on="Ring" class="Ring (strict)"() -> ("Strings []"=w391:string[])  [unwired: 2 in, 2 out]
        n257 = Index Array(array=w391, index=w390) -> (element=w389:string)
        n258 = call <vilib>:"NT Write String.vi"("String"=w389, "Name"=w388) -> ()  [unwired: 9 in, 1 out]
      }
    }
  }
  n259 = Index Array(array=w13) -> (element=w14:cluster{string[]})  [unwired: 1 in]
  n260 = Unbundle(w14) -> (w12:string[])
  n261 = Match First String(2:w12, 3:w11) -> (0:w10:i32)  [unwired: 1 out]
  n262 = Bundle("value"=w16, "value"=w15, "index"=w10) -> (w4:cluster{"value":i32, "value":i32, "index":i32})  [unwired: 1 out]
  n263 = property on="On/Off" class="Bool (strict)"("Visible"=w27) -> ()  [unwired: 2 in, 2 out]
  n264 = property on="Camera Settings" class="Clust (strict)"("Val(Sgnl)"=w4) -> ()  [unwired: 2 in, 2 out]
  n265 = property on="Motor" class="Clust (strict)"("Visible"=w27) -> ()  [unwired: 2 in, 2 out]
  n266 = property on="Progress" class="Clust (strict)"("Visible"=w27) -> ()  [unwired: 2 in, 2 out]
  n267 = property on="Ring" class="Ring (strict)"("Visible"=w27) -> ()  [unwired: 2 in, 2 out]
  n268 = property on="Rev/Fwd" class="Clust (strict)"("Visible"=w27) -> ()  [unwired: 2 in, 2 out]
  n269 = local write "DB Camera Config"(w27) -> ()
  n270 = property on="Camera Settings" class="Clust (strict)"("Visible"=w27) -> ()  [unwired: 2 in, 2 out]
